vi "setError.vi"(1 "error":errorcluster) -> ()   [LabVIEW 2010]
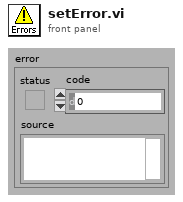
[diagram p1: front panel]
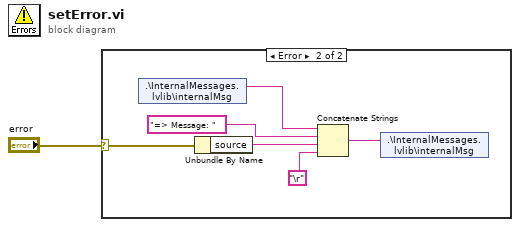
[diagram p0: block diagram]
diagram:
  n1 = case shown="Error" "error" {
    selector: "error" -> [_ w7]
    frame No Error {
    }
    frame Error {
      n2 = shared-variable ".\\InternalMessages.lvlib\\internalMsg"() -> (w3:string)  [unwired: 2 out]
      n3 = Unbundle By Name(w7) -> ("source"=w5:string)
      n4 = Concatenate Strings(w3, "=> Message: " ("string"), w5, "\r") -> (w2:string)
      n5 = shared-variable ".\\InternalMessages.lvlib\\internalMsg"(w2) -> ()  [unwired: 2 out]
    }
  }
